vi "Range_selector.vi"(11 "current":dbl) -> (3 "range integer":i32)   [LabVIEW 2022 SP3]
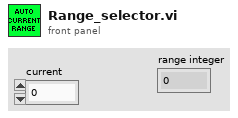
[diagram p1: front panel]
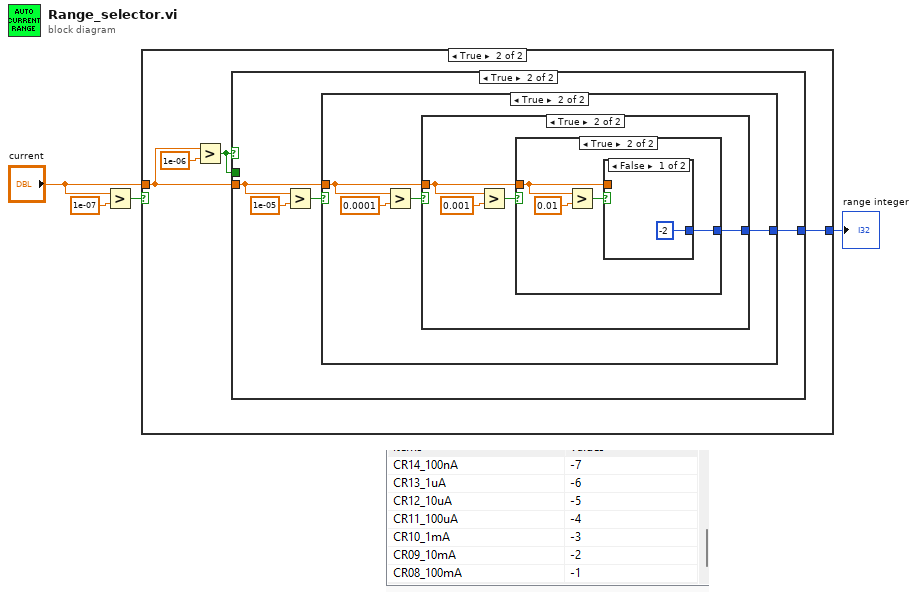
[diagram p0: block diagram]
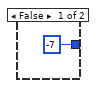
[diagram p2: hidden frame]
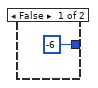
[diagram p3: hidden frame]
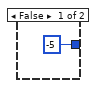
[diagram p4: hidden frame]
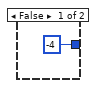
[diagram p5: hidden frame]
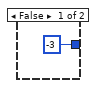
[diagram p6: hidden frame]
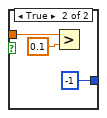
[diagram p7: hidden frame]
diagram:
  n1 = Greater?(x="current", y=1e-07) -> (0:w3:bool)
  n2 = case shown="True" w3 {
    tunnel: "current" -> [_ w8]
    tunnel: [-7 w6] -> w1
    frame False {
    }
    frame True {
      n3 = Greater?(x=w8, y=1e-06) -> (0:w7:bool)
      n4 = case shown="True" w7 {
        tunnel: w7 -> [_ _]
        tunnel: w8 -> [_ w12]
        tunnel: [-6 w11] -> w6
        frame False {
        }
        frame True {
          n5 = Greater?(x=w12, y=1e-05) -> (0:w13:bool)
          n6 = case shown="True" w13 {
            tunnel: w12 -> [_ w17]
            tunnel: [-5 w16] -> w11
            frame False {
            }
            frame True {
              n7 = Greater?(x=w17, y=0.0001) -> (0:w18:bool)
              n8 = case shown="True" w18 {
                tunnel: w17 -> [_ w22]
                tunnel: [-4 w21] -> w16
                frame False {
                }
                frame True {
                  n9 = Greater?(x=w22, y=0.001) -> (0:w23:bool)
                  n10 = case shown="True" w23 {
                    tunnel: w22 -> [_ w27]
                    tunnel: [-3 w26] -> w21
                    frame False {
                    }
                    frame True {
                      n11 = Greater?(x=w27, y=0.01) -> (0:w28:bool)
                      n12 = case shown="False" w28 {
                        tunnel: w27 -> [_ w32]
                        tunnel: [-2 -1] -> w26
                        frame False {
                        }
                        frame True {
                          n13 = Greater?(x=w32, y=0.1) -> ()  [unwired: 1 out]
                        }
                      }
                    }
                  }
                }
              }
            }
          }
        }
      }
    }
  }
  "range integer" <- w1
